vi "_toml_example2.vi"() -> ()   [LabVIEW 2017]
uses:
  b840e024-a058-4075-b0d4-c9d64e0cf193.vi
  toml_value_boolean.vi
panel:
  out "error out":errorcluster
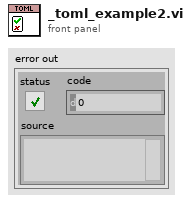
[diagram p1: front panel]
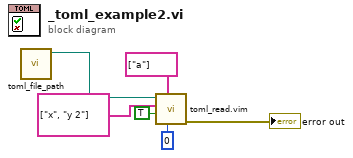
[diagram p0: block diagram]
diagram:
  n1 = call "toml_file_path.vi"() -> ("app toml path"=w5:path)  [unwired: 8 in, 3 out]
  n2 = call "toml_read.vim"("modifiers"=u16 0, "section [str,1d,pth]"=string[] ["a"] ("section"), "default [any]"=TRUE ("default"), "key [str,1d,pth]"=string[] ["x", "y 2"] ("key"), "path in"=w5) -> ("error out"=→"error out":errorcluster)  [unwired: 3 in, 3 out]
